vi "DBM Insert Data.vi"(4 "Slide 참조 번호":refnum<vi>, 5 "Query info":T1, 6 "배열":refnum<vi>[](array[refnum]), 7 "데이터":T3, 8 "에러 입력":errorcluster caption="에러 입력(에러 없음)", 11 "참조 번호 입력":T2) -> (0 "에러 출력":errorcluster, 3 "참조 번호 출력":T2)   [LabVIEW 2020]
uses:
  <vilib>/addons/database/Connection.llb/Conn ObjectReference.ctl
  Controls/Clst_DBM data.ctl
  Controls/Clst_Query Info.ctl
  Controls/Cmd_Read Query.ctl
  Controls/Cmd_Write Query.ctl
  Public/Polymorph/Rmv Empt Arr_2D Str.vi
  <vilib>/addons/database/NI_Database_API.lvlib
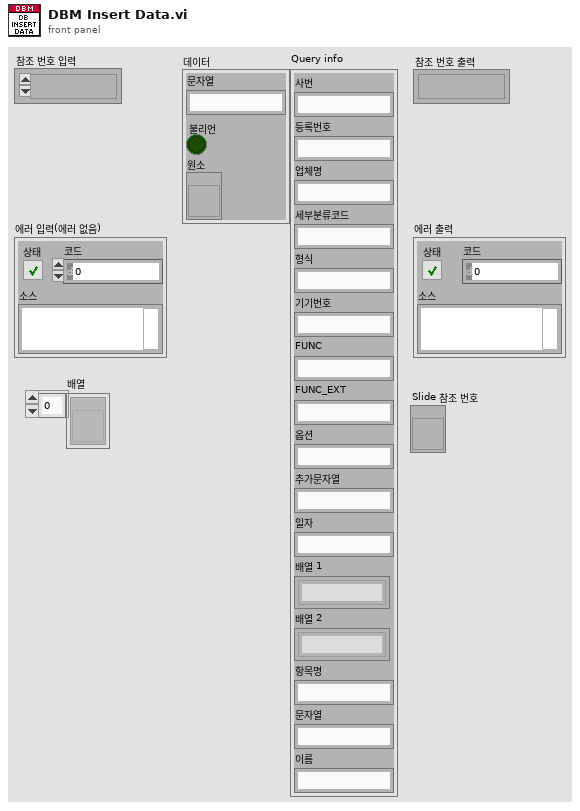
[diagram p1: front panel]
types:
  T1 = typedef "Clst_Query Info.ctl" = cluster{"사번":string, "등록번호":string, "업체명":string, "세부분류코드":string, "형식":string, "기기번호":string, "FUNC":string, "FUNC_EXT":string, "옵션":string, "추가문자열":string, "일자":string, "배열 1":string[], "배열 2":string[], "항목명":string, "문자열":string, "이름":string}
  T2 = typedef "NI_Database_API.lvlib/Conn ObjectReference.ctl" = refnum<k1>
  T3 = typedef "Clst_DBM data.ctl" = cluster{"문자열":string, "불리언":bool, "원소":refnum<vi>}
  T4 = typedef "Cmd_Read Query.ctl" = enum16{"교정자 이름 얻기", "인증교정자 얻기", "기술책임자 얻기", "기책부책 얻기", "등록번호 얻기", "등록정보 얻기", "업체정보 얻기", "교정일자(CAMAS) 얻기", "교정일자(CALSTD) 얻기", "교정환경 얻기", "교정절차서 목록 얻기", "교정절차서명 얻기", "교정절차 목록얻기", "교정절차 얻기", "PROC 교정절차 얻기", "PROC SPEC 얻기", "교정절차(Func별) 얻기", "교정절차(Func_ext별) 얻기", "기관코드 얻기", "교정기능(세부분류) 얻기", "교정기능(모델) 얻기", "교정기능 목록 얻기", "교정기능 명칭 얻기", "교정기능 항목명칭 얻기", "DB (사용기준기) 얻기", "DB (기준기이름) 얻기", "DB (기준기이름목록) 얻기", "DB (기준기목록) 얻기", "DB (기준기값) 얻기", "DB (CMC) 얻기", "DB (FUNC) 얻기", "DB (CALNAME) 얻기", "DB (STDNAME) 얻기", "DB (SPEC) 얻기", "모델(항목전체) 얻기", "모델(최대범위) 얻기", "모델(최소범위) 얻기", "모델(최대최소) 얻기", "모델(범위조건) 얻기", "모델(등록요청) 얻기", "모델(형식별) 얻기", "모델(조건별) 얻기", "모델(모델검색) 얻기", "세부분류 목록 얻기", "기준기등록리스트 얻기", "STD Cal Date Check", "DB등록일자 얻기", "적용항목 얻기", "기타정보 얻기", "기준기요청 얻기", "서버버전 얻기"}
  T5 = typedef "Cmd_Write Query.ctl" = enum16{"TBUSESTD_MCT Insert", "TBUSESTD_MCT Delete", "TBCALSTD_MCT_TEMP Insert", "TBCALSTD_MCT_TEMP Delete", "TBCALSTD_MCT Insert", "TBCALSTD_MCT Delete", "TBCALSTD_MCT_BACK Insert", "TBCALSTD_MCT_BACK Delete", "TBCALPROC_MCT Insert", "TBCALPROC_MCT Delete", "TBCALPROC_MCT_TEMP Insert", "TBCALPROC_MCT_TEMP Delete", "TBCALCMC_MCT Insert", "TBCALCMC_MCT Delete", "TBCALFUNC_MCT Insert", "TBCALFUNC_MCT Delete", "TBCALNAME_MCT Insert", "TBCALNAME_MCT Delete", "TBSTDNAME_MCT Insert", "TBSTDNAME_MCT Delete", "TBCALSPEC_MCT Insert", "TBCALSPEC_MCT Delete", "TBCALSTD_MCT NOTUSE update", "TBCALSPEC_MCT update", "TBMCTVERMAN update"}
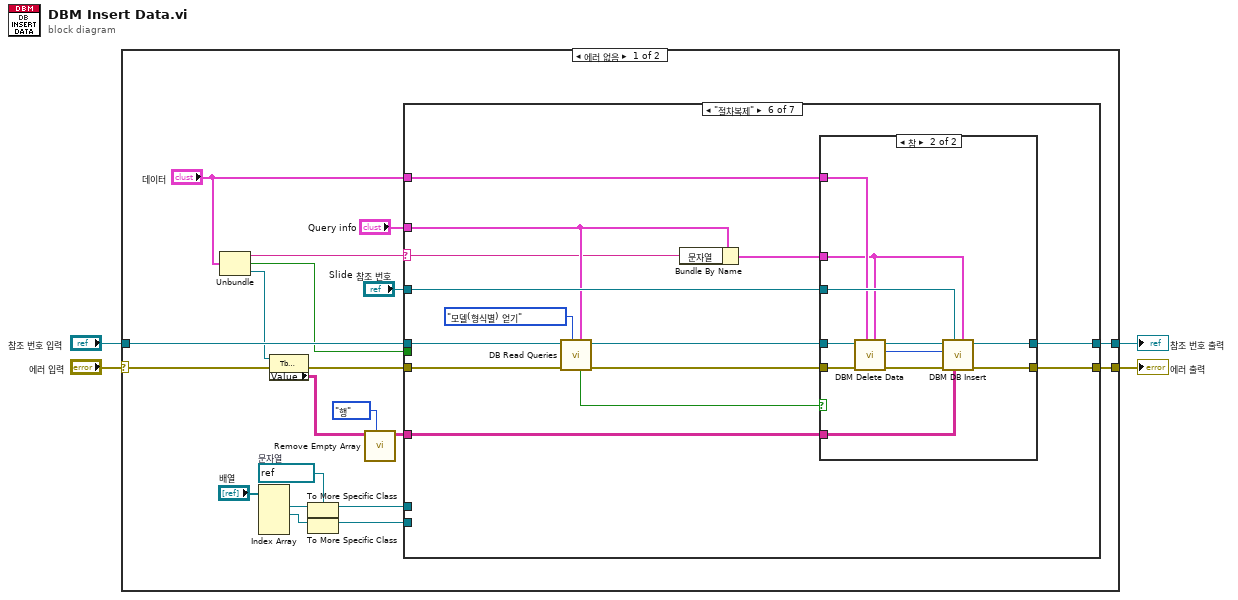
[diagram p0: block diagram]
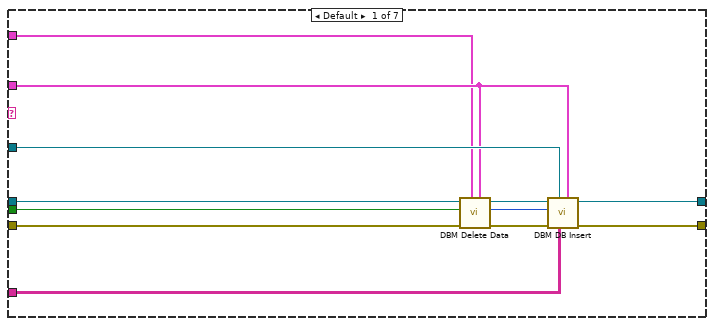
[diagram p2: hidden frame]
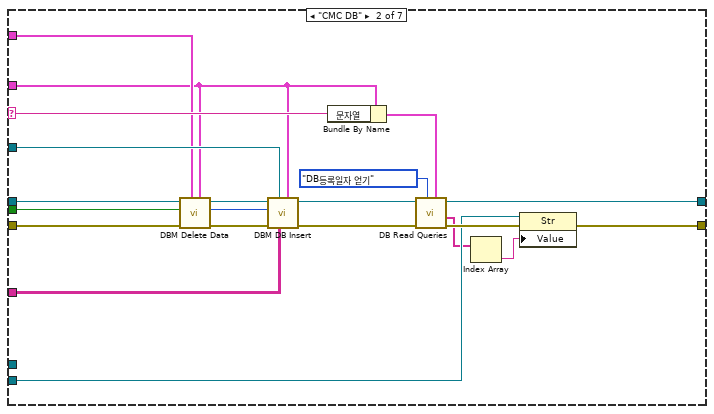
[diagram p3: hidden frame]
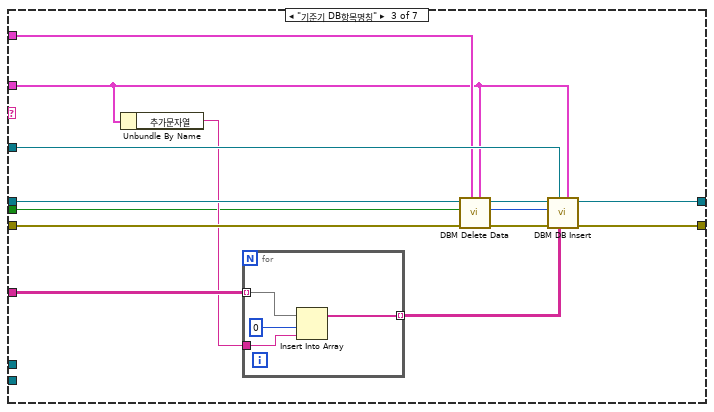
[diagram p4: hidden frame]
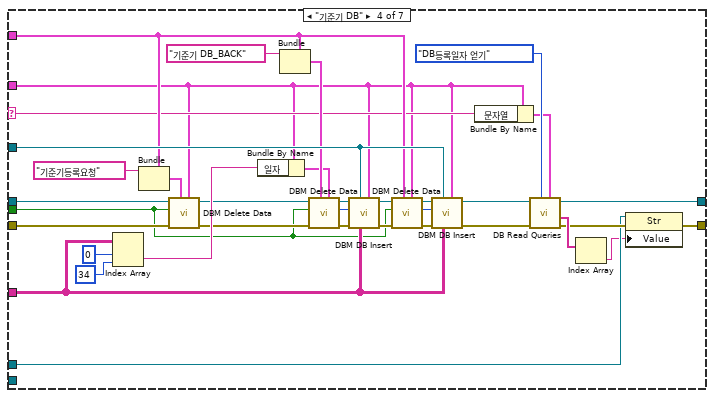
[diagram p5: hidden frame]
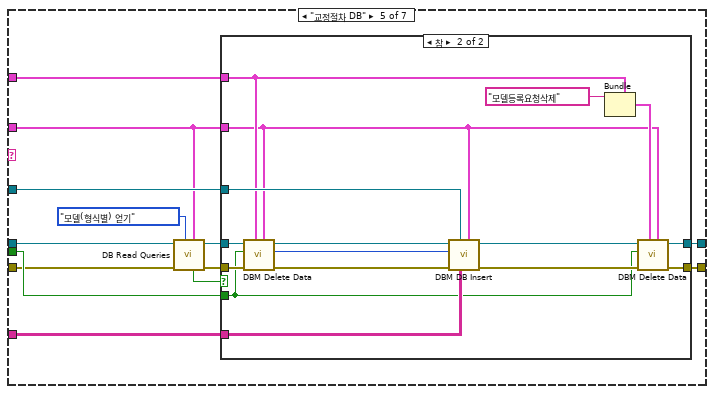
[diagram p6: hidden frame]
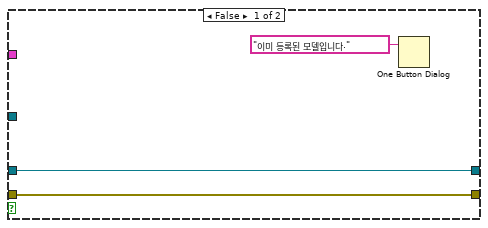
[diagram p7: hidden frame]
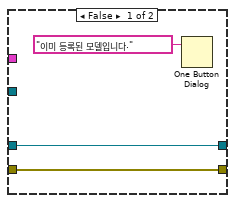
[diagram p8: hidden frame]
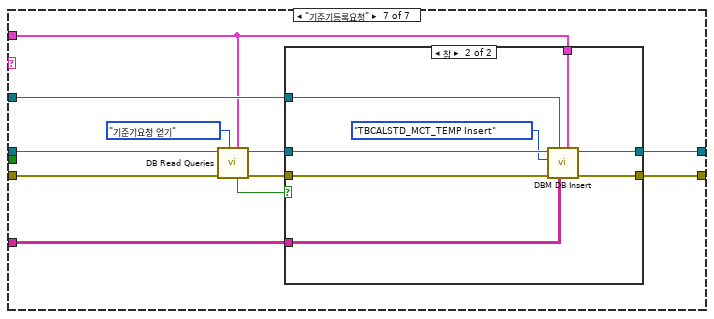
[diagram p9: hidden frame]
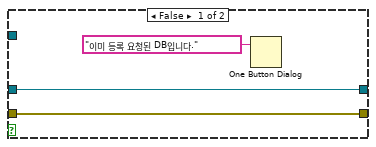
[diagram p10: hidden frame]
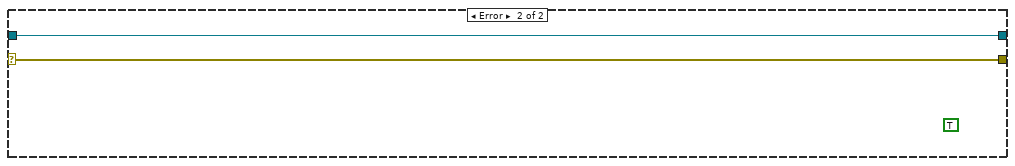
[diagram p11: hidden frame]
diagram:
  n1 = case shown="에러 없음" "에러 입력" {
    selector: "에러 입력" -> [w21 w195]
    tunnel: [w24 w195] -> w4
    tunnel: "참조 번호 입력" -> [w23 w194]
    tunnel: [w22 w194] -> w2
    frame No Error {
      w14 = refnum<vi> refnum  # 문자열
      n2 = Unbundle("데이터") -> ("문자열"=w10:string, "불리언"=w7:bool, "원소"=w6:refnum<vi>)
      n3 = Index Array(array="배열") -> (element #1=w18:refnum<vi>, element #2=w16:refnum<vi>)  [unwired: 4 in, 2 out]
      n4 = property class="Tbl (엄격한)"(reference=w6, error in=w21) -> (error out=w20:errorcluster, "Value"=w13:string[][])  [unwired: 1 out]
      n5 = To More Specific Class(target class=w14, reference=w18) -> (specific class reference=w17:refnum<vi>)  [unwired: 1 in, 1 out]
      n6 = To More Specific Class(target class=w14, reference=w16) -> (specific class reference=w15:refnum<vi>)  [unwired: 1 in, 1 out]
      n7 = call-poly "Remove Empty Array.vi"("조건"=enum16{"행", "열", "행,열"}."행", "Data in"=w13) -> ("Data out"=w11:string[][])  [unwired: 8 in, 1 out]
      n8 = case shown="\"절차복제\"" w10 {
        selector: w10 -> [_ w46 _ w77 _ w145 _]
        tunnel: w20 -> [w35 w56 w70 w87 w113 w154 w178]
        tunnel: [w32 w43 w67 w90 w118 w150 w182] -> w24
        tunnel: "Query info" -> [w26 w37 w58 w76 w114 w146 w174]
        tunnel: w23 -> [w36 w57 w71 w88 w122 w155 w173]
        tunnel: [w31 w49 w66 w96 w117 w149 w181] -> w22
        tunnel: "데이터" -> [w25 w38 w59 w78 w119 w151 _]
        tunnel: "Slide 참조 번호" -> [w30 w53 w65 w103 w116 w148 w180]
        tunnel: w11 -> [w29 w52 w63 w99 w112 w147 w179]
        tunnel: w17 -> [_ _ _ w91 _ _ _]
        tunnel: w15 -> [_ w42 _ _ _ _ _]
        tunnel: w7 -> [w27 w39 w60 w82 w115 _ _]
        frame Default {
          n9 = call "DBM Delete Data.vi"("Query info"=w26, "데이터"=w25, "에러 입력"=w35, "추가?"=w27, "참조 번호 입력"=w36) -> ("에러 출력"=w33:errorcluster, "COMMAND"=w28:T5, "참조 번호 출력"=w34:T2)  [unwired: 4 in]
          n10 = call "DBM DB Insert.vi"("Query info"=w26, "Value"=w29, "Slide 입력"=w30, "에러 입력"=w33, "COMMAND"=w28, "참조 번호 입력"=w34) -> ("에러 출력"=w32:errorcluster, "참조 번호 출력"=w31:T2)  [unwired: 4 in]
        }
        frame "CMC DB" {
          n11 = call "DBM Delete Data.vi"("Query info"=w37, "데이터"=w38, "에러 입력"=w56, "추가?"=w39, "참조 번호 입력"=w57) -> ("에러 출력"=w54:errorcluster, "COMMAND"=w51:T5, "참조 번호 출력"=w55:T2)  [unwired: 4 in]
          n12 = call "DBM DB Insert.vi"("Query info"=w37, "Value"=w52, "Slide 입력"=w53, "에러 입력"=w54, "COMMAND"=w51, "참조 번호 입력"=w55) -> ("에러 출력"=w48:errorcluster, "참조 번호 출력"=w50:T2)  [unwired: 4 in]
          n13 = Bundle By Name(cluster=w37, "문자열"=w46) -> (w45:T1)
          n14 = call "DB Read Queries.vi"("Query info"=w45, "Query Command"=Cmd_Read_Query."DB등록일자 얻기", "에러 입력(에러 없음)"=w48, "참조 번호 입력"=w50) -> ("에러 출력"=w44:errorcluster, "Data (0번행)"=w41:string[], "참조 번호 출력"=w49:T2)  [unwired: 3 in, 2 out]
          n15 = Index Array(array=w41) -> (element=w40:string)  [unwired: 1 in]
          n16 = property class="Str"(reference=w42, error in=w44, "Value"=w40) -> (error out=w43:errorcluster)  [unwired: 1 out]
        }
        frame "기준기 DB항목명칭" {
          n17 = Unbundle By Name(w58) -> ("추가문자열"=w62:string)
          n18 = for {
            tunnel: w63 -> [w75] mode=indexing
            tunnel: w62 -> [w74]
            tunnel: [w72] -> w61 mode=indexing
            n19 = Insert Into Array(array=w75, index=0 ("인덱스"), new element=w74) -> (w72:string[])
          }
          n20 = call "DBM Delete Data.vi"("Query info"=w58, "데이터"=w59, "에러 입력"=w70, "추가?"=w60, "참조 번호 입력"=w71) -> ("에러 출력"=w68:errorcluster, "COMMAND"=w64:T5, "참조 번호 출력"=w69:T2)  [unwired: 4 in]
          n21 = call "DBM DB Insert.vi"("Query info"=w58, "Value"=w61, "Slide 입력"=w65, "에러 입력"=w68, "COMMAND"=w64, "참조 번호 입력"=w69) -> ("에러 출력"=w67:errorcluster, "참조 번호 출력"=w66:T2)  [unwired: 4 in]
        }
        frame "기준기 DB" {
          n22 = Index Array(array=w99, index (row)=0 ("인덱스 (행)"), index (col)=34 ("비활성화된 인덱스 (열)")) -> (element=w100:string)
          n23 = Bundle(cluster=w78, "문자열"="기준기등록요청") -> (w81:T3)  [unwired: 2 in]
          n24 = call "DBM Delete Data.vi"("Query info"=w76, "데이터"=w81, "에러 입력"=w87, "추가?"=w82, "참조 번호 입력"=w88) -> ("에러 출력"=w86:errorcluster, "참조 번호 출력"=w85:T2)  [unwired: 4 in, 1 out]
          n25 = Bundle By Name(cluster=w76, "일자"=w100) -> (w79:T1)
          n26 = Bundle(cluster=w78, "문자열"="기준기 DB_BACK") -> (w80:T3)  [unwired: 2 in]
          n27 = call "DBM Delete Data.vi"("Query info"=w79, "데이터"=w80, "에러 입력"=w86, "추가?"=w82, "참조 번호 입력"=w85) -> ("에러 출력"=w107:errorcluster, "COMMAND"=w108:T5, "참조 번호 출력"=w106:T2)  [unwired: 4 in]
          n28 = call "DBM DB Insert.vi"("Query info"=w76, "Value"=w99, "Slide 입력"=w103, "에러 입력"=w107, "COMMAND"=w108, "참조 번호 입력"=w106) -> ("에러 출력"=w105:errorcluster, "참조 번호 출력"=w104:T2)  [unwired: 4 in]
          n29 = call "DBM Delete Data.vi"("Query info"=w76, "데이터"=w78, "에러 입력"=w105, "추가?"=w82, "참조 번호 입력"=w104) -> ("에러 출력"=w110:errorcluster, "COMMAND"=w109:T5, "참조 번호 출력"=w111:T2)  [unwired: 4 in]
          n30 = call "DBM DB Insert.vi"("Query info"=w76, "Value"=w99, "Slide 입력"=w103, "에러 입력"=w110, "COMMAND"=w109, "참조 번호 입력"=w111) -> ("에러 출력"=w97:errorcluster, "참조 번호 출력"=w98:T2)  [unwired: 4 in]
          n31 = Bundle By Name(cluster=w76, "문자열"=w77) -> (w93:T1)
          n32 = call "DB Read Queries.vi"("Query info"=w93, "Query Command"=Cmd_Read_Query."DB등록일자 얻기", "에러 입력(에러 없음)"=w97, "참조 번호 입력"=w98) -> ("에러 출력"=w92:errorcluster, "Data (0번행)"=w94:string[], "참조 번호 출력"=w96:T2)  [unwired: 3 in, 2 out]
          n33 = Index Array(array=w94) -> (element=w89:string)  [unwired: 1 in]
          n34 = property class="Str"(reference=w91, error in=w92, "Value"=w89) -> (error out=w90:errorcluster)  [unwired: 1 out]
        }
        frame "교정절차 DB" {
          n35 = call "DB Read Queries.vi"("Query info"=w114, "Query Command"=Cmd_Read_Query."모델(형식별) 얻기", "에러 입력(에러 없음)"=w113, "참조 번호 입력"=w122) -> ("에러 출력"=w121:errorcluster, "참조 번호 출력"=w120:T2, "None?"=w123:bool)  [unwired: 3 in, 2 out]
          n36 = case shown="참" w123 {
            tunnel: w121 -> [w127 w143]
            tunnel: w120 -> [w126 w142]
            tunnel: w119 -> [_ w129]
            tunnel: [w127 w136] -> w118
            tunnel: [w126 w134] -> w117
            tunnel: w116 -> [_ w139]
            tunnel: w112 -> [_ w138]
            tunnel: w115 -> [_ w130]
            tunnel: w114 -> [_ w128]
            frame False {
              n37 = One Button Dialog(message="이미 등록된 모델입니다." ("메시지")) -> ()  [unwired: 1 in, 1 out]
            }
            frame True {
              n38 = call "DBM Delete Data.vi"("Query info"=w128, "데이터"=w129, "에러 입력"=w143, "추가?"=w130, "참조 번호 입력"=w142) -> ("에러 출력"=w133:errorcluster, "COMMAND"=w140:T5, "참조 번호 출력"=w141:T2)  [unwired: 4 in]
              n39 = call "DBM DB Insert.vi"("Query info"=w128, "Value"=w138, "Slide 입력"=w139, "에러 입력"=w133, "COMMAND"=w140, "참조 번호 입력"=w141) -> ("에러 출력"=w137:errorcluster, "참조 번호 출력"=w135:T2)  [unwired: 4 in]
              n40 = Bundle(cluster=w129, "문자열"="모델등록요청삭제") -> (w132:T3)  [unwired: 2 in]
              n41 = call "DBM Delete Data.vi"("Query info"=w128, "데이터"=w132, "에러 입력"=w137, "추가?"=w130, "참조 번호 입력"=w135) -> ("에러 출력"=w136:errorcluster, "참조 번호 출력"=w134:T2)  [unwired: 4 in, 1 out]
            }
          }
        }
        frame "절차복제" {
          n42 = call "DB Read Queries.vi"("Query info"=w146, "Query Command"=Cmd_Read_Query."모델(형식별) 얻기", "에러 입력(에러 없음)"=w154, "참조 번호 입력"=w155) -> ("에러 출력"=w153:errorcluster, "참조 번호 출력"=w152:T2, "None?"=w156:bool)  [unwired: 3 in, 2 out]
          n43 = Bundle By Name(cluster=w146, "문자열"=w145) -> (w144:T1)
          n44 = case shown="참" w156 {
            tunnel: w153 -> [w160 w171]
            tunnel: w152 -> [w159 w170]
            tunnel: w151 -> [_ w162]
            tunnel: w144 -> [_ w161]
            tunnel: [w160 w168] -> w150
            tunnel: [w159 w167] -> w149
            tunnel: w148 -> [_ w164]
            tunnel: w147 -> [_ w163]
            frame False {
              n45 = One Button Dialog(message="이미 등록된 모델입니다." ("메시지")) -> ()  [unwired: 1 in, 1 out]
            }
            frame True {
              n46 = call "DBM Delete Data.vi"("Query info"=w161, "데이터"=w162, "에러 입력"=w171, "참조 번호 입력"=w170) -> ("에러 출력"=w169:errorcluster, "COMMAND"=w165:T5, "참조 번호 출력"=w166:T2)  [unwired: 5 in]
              n47 = call "DBM DB Insert.vi"("Query info"=w161, "Value"=w163, "Slide 입력"=w164, "에러 입력"=w169, "COMMAND"=w165, "참조 번호 입력"=w166) -> ("에러 출력"=w168:errorcluster, "참조 번호 출력"=w167:T2)  [unwired: 4 in]
            }
          }
        }
        frame "기준기등록요청" {
          n48 = call "DB Read Queries.vi"("Query info"=w174, "Query Command"=Cmd_Read_Query."기준기요청 얻기", "에러 입력(에러 없음)"=w178, "참조 번호 입력"=w173) -> ("에러 출력"=w177:errorcluster, "참조 번호 출력"=w172:T2, "None?"=w175:bool)  [unwired: 3 in, 2 out]
          n49 = case shown="참" w175 {
            tunnel: w172 -> [w184 w193]
            tunnel: w174 -> [_ w192]
            tunnel: [w185 w191] -> w182
            tunnel: [w184 w190] -> w181
            tunnel: w180 -> [_ w189]
            tunnel: w179 -> [_ w188]
            tunnel: w177 -> [w185 w186]
            frame False {
              n50 = One Button Dialog(message="이미 등록 요청된 DB입니다." ("메시지")) -> ()  [unwired: 1 in, 1 out]
            }
            frame True {
              n51 = call "DBM DB Insert.vi"("Query info"=w192, "Value"=w188, "Slide 입력"=w189, "에러 입력"=w186, "COMMAND"=Cmd_Write_Query."TBCALSTD_MCT_TEMP Insert", "참조 번호 입력"=w193) -> ("에러 출력"=w191:errorcluster, "참조 번호 출력"=w190:T2)  [unwired: 4 in]
            }
          }
        }
      }
    }
    frame Error {
      (unwired) TRUE ("에러?")
    }
  }
  "에러 출력" <- w4
  "참조 번호 출력" <- w2
